vi "Get RSSI.vi"(8 "error in (no error)":errorcluster caption="entrée d'erreur (pas d'erreur)", 11 "Parsing Data RADIO_ERP1 en entrée":refnum<class "Parsing Data RADIO_ERP1.lvclass">) -> (0 "error out":errorcluster caption="sortie d'erreur", 2 "RSSI":string, 3 "Parsing Data RADIO_ERP1 en sortie":refnum<class "Parsing Data RADIO_ERP1.lvclass">)   [LabVIEW 2020, in "Library Instrument & Equipement.lvlib" / "Library UART.lvlib" / "Parsing Data RADIO_ERP1.lvclass"]
uses:
  Parsing Data RADIO_ERP1.lvclass
  Parsing Data RADIO_ERP1.lvclass/Parsing Data RADIO_ERP1.ctl
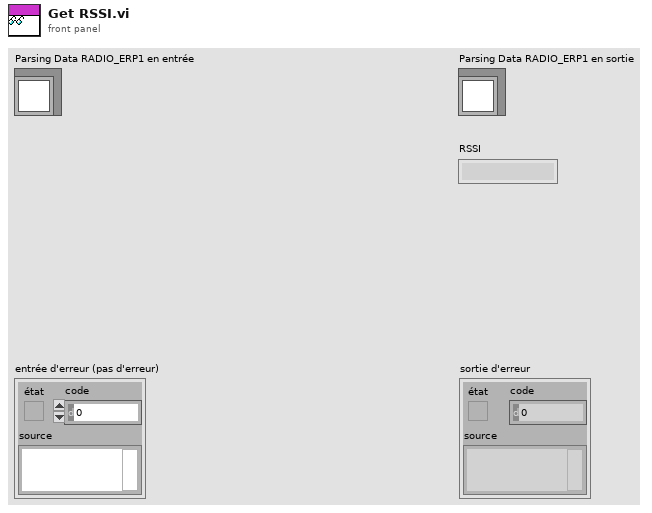
[diagram p1: front panel]
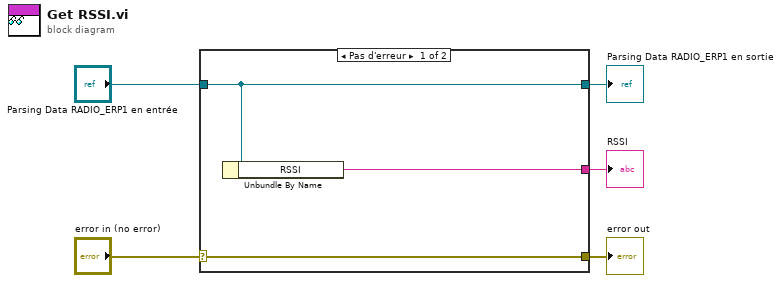
[diagram p0: block diagram]
diagram:
  n1 = case shown="Pas d'erreur" "error in (no error)" {
    selector: "error in (no error)" -> [w8 w9]
    tunnel: [w8 w9] -> w4
    tunnel: [w7 w10] -> w2
    tunnel: "Parsing Data RADIO_ERP1 en entrée" -> [w7 w10]
    tunnel: [w6 _] -> w1
    frame No Error {
      n2 = Unbundle By Name(w7) -> ("RSSI"=w6:string)
    }
    frame Error {
    }
  }
  "error out" <- w4
  "Parsing Data RADIO_ERP1 en sortie" <- w2
  "RSSI" <- w1
